vi "AddErrorCase__slk_mt.vi"(8 "error in (no error)":errorcluster, 10 "vi name":string, 11 "application reference":refnum<vi>) -> (0 "error out":errorcluster)   [LabVIEW 2010, in "Lazyboots Menu Tool.lvlib"]
doc: "This VI is the core of <b>Add Error Case</b> function, and will be called by corresponding menu launcher."
uses:
  Library/Lazyboots Menu Tool.lvlib
  Private/AddErrorCase/TypeDef/TypeDef_AddErrorCaseState__slk_mt.ctl
  <vilib>/Utility/config.llb/NI_LVConfig.lvlib
panel:
  # "AddErrorCase__slk_mt.vi\nThis VI is the core of <b>Add Error Case</b> function, and will be called by corresponding menu launcher.\n\nNOTICE -- YOU MUST LEAVE THIS NOTICE IN PLACE.\n\nCopyright (c) 2011, LIANG LIU Shawn.Liu.cn@gmail.com\nAll rights reserved.\n\nRedistribution and use in source and binary forms, with or without modification, are permitted provided that the following conditions are met:\n-Redistributions of source code must retain the above copyright notice, this list of conditions and the following disclaimer.\n-Redistributions in binary form must reproduce the above copyright notice, this list of conditions and the following disclaimer in the documentation and/or other materials provided with the distribution.\n-Neither the name of the eLp nor the names of its contributors may be used to endorse or promote products derived from this software without specific prior written permission.\n\nTHIS SOFTWARE IS PROVIDED BY THE COPYRIGHT HOLDERS AND CONTRIBUTORS \"AS IS\" AND ANY EXPRESS OR IMPLIED WARRANTIES, INCLUDING, BUT NOT LIMITED TO, THE IMPLIED WARRANTIES OF MERCHANTABILITY AND FITNESS FOR A PARTICULAR PURPOSE ARE DISCLAIMED. IN NO EVENT SHALL THE COPYRIGHT HOLDER OR CONTRIBUTORS BE LIABLE FOR ANY DIRECT, INDIRECT, INCIDENTAL, SPECIAL, EXEMPLARY, OR CONSEQUENTIAL DAMAGES (INCLUDING, BUT NOT LIMITED TO, PROCUREMENT OF SUBSTITUTE GOODS OR SERVICES; LOSS OF USE, DATA, OR PROFITS; OR BUSINESS INTERRUPTION) HOWEVER CAUSED AND ON ANY THEORY OF LIABILITY, WHETHER IN CONTRACT, STRICT LIABILITY, OR TORT (INCLUDING NEGLIGENCE OR OTHERWISE) ARISING IN ANY WAY OUT OF THE USE OF THIS SOFTWARE, EVEN IF ADVISED OF THE POSSIBILITY OF SUCH DAMAGE."
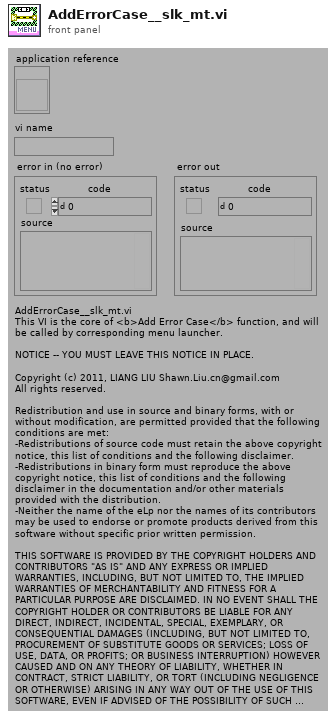
[diagram p1: front panel]
types:
  T1 = typedef "Lazyboots Menu Tool.lvlib/TypeDef_AddErrorCaseState__slk_mt.ctl" = enum16{"Read Configure", "Get Menu Launch VI", "Undo.Start", "Add Error Case", "Undo.End/Fail", "End"}
  T2 = typedef "NI_LVConfig.lvlib/Config Data RefNum.ctl" = refnum<k1>
  T3 = typedef "Lazyboots Menu Tool.lvlib/TypeDef_AddErrorCaseConfigure__slk_mt.ctl" = cluster{"Frame Width":u32, "Create Constant":bool}
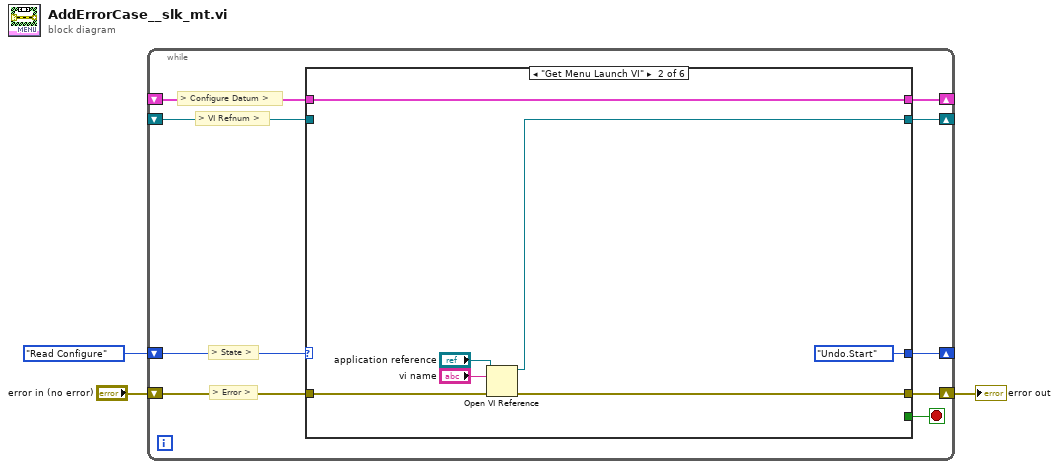
[diagram p0: block diagram]
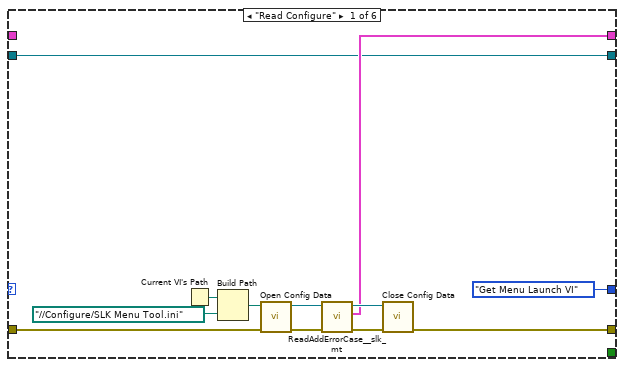
[diagram p2: hidden frame]
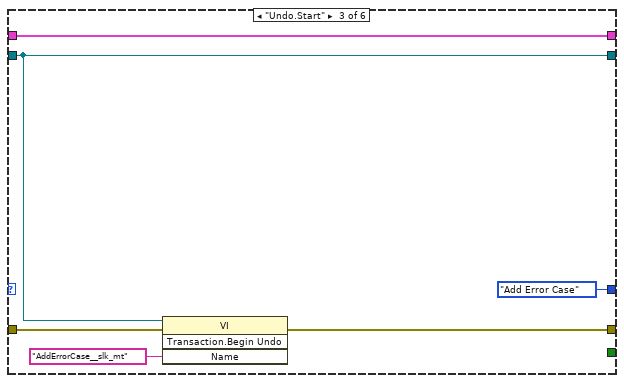
[diagram p3: hidden frame]
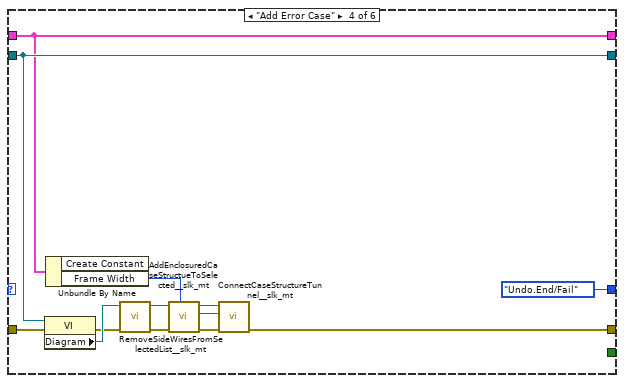
[diagram p4: hidden frame]
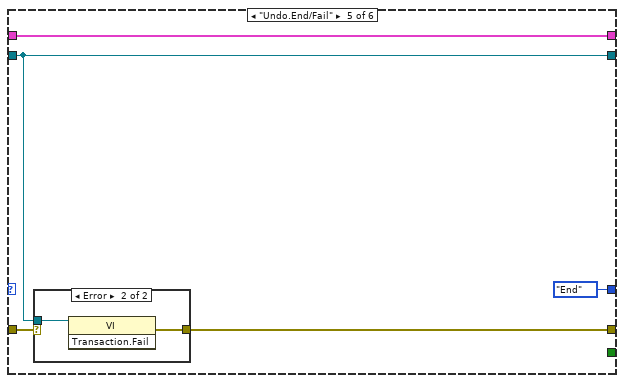
[diagram p5: hidden frame]
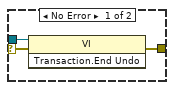
[diagram p6: hidden frame]
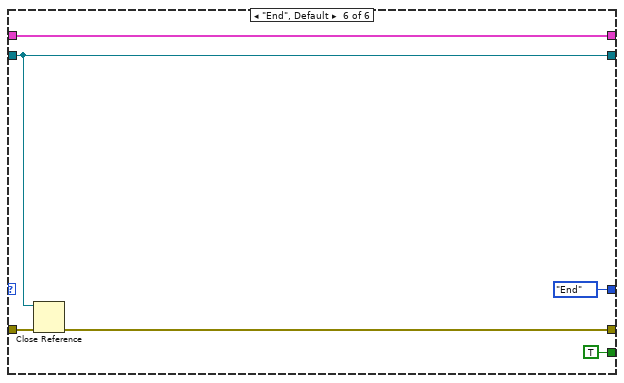
[diagram p7: hidden frame]
diagram:
  n1 = while {
    shift-right: [w9] -> _
    shift-left: TypeDef_AddErrorCaseState__slk_mt."Read Configure" ("State") -> [w12]
    shift-right: [w10] -> w1
    shift-left: "error in (no error)" -> [w11]
    shift-right: [w7] -> _
    shift-left: _ -> [w8]
    shift-right: [w5] -> _
    shift-left: _ -> [w6]
    stop <- w4 stop-if-true
    # "> VI Refnum >"
    # "> Configure Datum >"
    # "> Error >"
    # "> State >"
    n2 = case shown="\"Get Menu Launch VI\"" w12 {
      tunnel: w11 -> [w18 w31 w36 w50 w53 w61]
      tunnel: [w16 w29 w35 w40 w52 w63] -> w10
      tunnel: [TypeDef_AddErrorCaseState__slk_mt."Get Menu Launch VI" ("State") TypeDef_AddErrorCaseState__slk_mt."Undo.Start" ("State") TypeDef_AddErrorCaseState__slk_mt."Add Error Case" ("State") TypeDef_AddErrorCaseState__slk_mt."Undo.End/Fail" ("State") TypeDef_AddErrorCaseState__slk_mt."End" ("State") TypeDef_AddErrorCaseState__slk_mt."End" ("State")] -> w9
      tunnel: w8 -> [_ w28 w37 w39 w55 w66]
      tunnel: [w14 w28 w37 w39 w55 w66] -> w7
      tunnel: w6 -> [w13 _ w34 w49 w51 w62]
      tunnel: [w13 w27 w34 w49 w51 w62] -> w5
      tunnel: [_ _ _ _ _ TRUE] -> w4
      frame "Read Configure" {
        n3 = Current VI's Path() -> (path=w20:path)
        n4 = Build Path(base path=w20, name or relative path=path "../../Configure/SLK Menu Tool.ini") -> (appended path=w19:path)
        n5 = call <vilib>:"Open Config Data.vi"("error in (no error)"=w18, "configuration file path"=w19) -> ("error out"=w23:errorcluster, "refnum"=w24:T2)  [unwired: 7 in, 1 out]
        n6 = call "ReadAddErrorCase__slk_mt.vi"("error in (no error)"=w23, "refnum in"=w24) -> ("error out"=w22:errorcluster, "add error case configure"=w14:T3, "refnum out"=w21:T2)  [unwired: 7 in]
        n7 = call <vilib>:"Close Config Data.vi"("error in (no error)"=w22, "refnum"=w21) -> ("error out"=w16:errorcluster)  [unwired: 8 in, 1 out]
      }
      frame "Get Menu Launch VI" {
        n8 = Open VI Reference(application reference (local)="application reference", vi path="vi name", error in (no error)=w31) -> (vi reference=w27:refnum<vi>, error out=w29:errorcluster)  [unwired: 3 out]
      }
      frame "Undo.Start" {
        n9 = invoke class="VI" method="Transaction.Begin Undo"(reference=w34, error in=w36, "Name"="AddErrorCase__slk_mt") -> (error out=w35:errorcluster)  [unwired: 1 in, 3 out]
      }
      frame "Add Error Case" {
        n10 = property class="VI"(reference=w49, error in=w50) -> (error out=w41:errorcluster, "Diagram"=w42:refnum<vi>)  [unwired: 1 out]
        n11 = Unbundle By Name(w39) -> ("Frame Width"=w38:u32)  [unwired: 1 out]
        n12 = call "RemoveSideWiresFromSelectedList__slk_mt.vi"("error in (no error)"=w41, "diagram refnum in"=w42) -> ("error out"=w43:errorcluster, "duplicated diagram refnum out"=w44:refnum<vi>)  [unwired: 8 in]
        n13 = call "AddEnclosuredCaseStructueToSelected__slk_mt.vi"("frame width (20)"=w38, "error in (no error)"=w43, "diagram refnum in"=w44) -> ("error out"=w45:errorcluster, "case structure refnum out"=w46:refnum<vi>, "duplicated diagram refnum out"=w47:refnum<vi>)  [unwired: 6 in]
        n14 = call "ConnectCaseStructureTunnel__slk_mt.vi"("error in (no error)"=w45, "case structure refnum in"=w46, "diagram refnum in"=w47) -> ("error out"=w40:errorcluster)  [unwired: 6 in, 2 out]
      }
      frame "Undo.End/Fail" {
        n15 = case shown="Error" w53 {
          selector: w53 -> [w57 _]
          tunnel: w51 -> [w58 w60]
          tunnel: [w56 w59] -> w52
          frame No Error {
            n16 = invoke class="VI" method="Transaction.End Undo"(reference=w58, error in=w57) -> (error out=w56:errorcluster)  [unwired: 1 in, 2 out]
          }
          frame Error {
            n17 = invoke class="VI" method="Transaction.Fail"(reference=w60) -> (error out=w59:errorcluster)  [unwired: 2 in, 2 out]
          }
        }
      }
      frame "End", Default {
        n18 = Close Reference(reference=w62, error in (no error)=w61) -> (error out=w63:errorcluster)
      }
    }
  }
  "error out" <- w1
